vi "Request and Wait for Response.vi"(5 "headers":string, 7 "timeout in ms (-1)":i32=-1, 8 "error in":errorcluster {"code" format="Error %.0f"}, 9 "payload":string, 10 "subject":string, 11 "NATS Client in":refnum<class "NATS Client.lvclass">) -> (0 "error out":errorcluster {"code" format="Error %.0f"}, 2 "time out":bool, 3 "nats message":T1)   [LabVIEW 2020, in "NATS Client.lvlib" / "NATS Client.lvclass"]
doc: "Publishes a message and waits for a response with a blocking call."
uses:
  NATS Client.lvclass
  NATS Client.lvclass/NATS Client.ctl
  NATS Subscription/NATS Subscription.lvclass/NATS Subscription.ctl
  <vilib>/NATS/NATS Core/NATS Core.lvlib
  NATS Subscription/NATS Subscription.lvclass
  <vilib>/NATS/NATS Core/VIs/NATS HPUB.vi
  <vilib>/NATS/NATS Core/Controls/msg type.ctl
  <vilib>/NATS/NATS Core/Controls/nats message.ctl
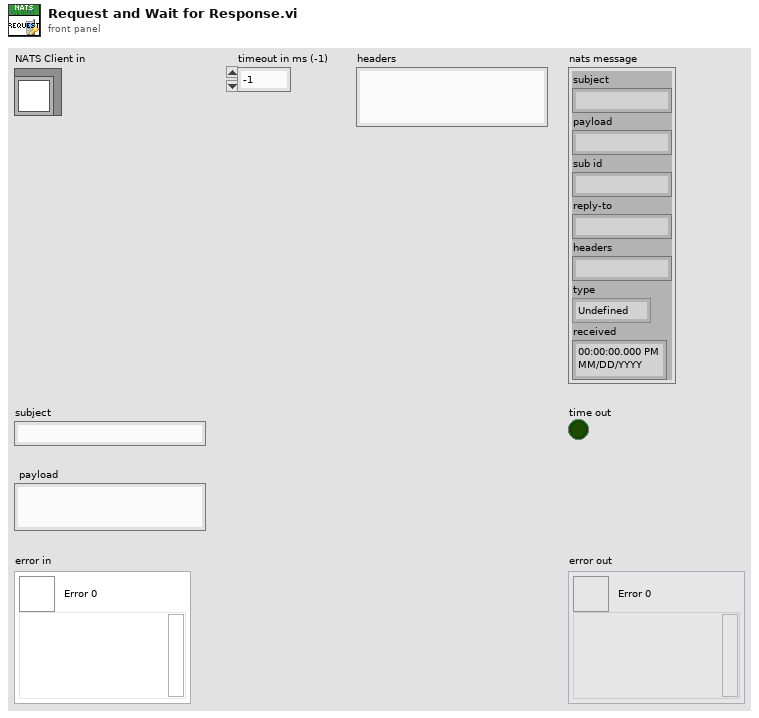
[diagram p1: front panel]
types:
  T1 = typedef "NATS Core.lvlib/nats message.ctl" = cluster{"subject":string, "payload":string, "sub id":string, "reply-to":string, "headers":string, "type":T2, "received":timestamp}
  T2 = typedef "NATS Core.lvlib/msg type.ctl" = enum16{"Undefined", "MSG", "HMSG", "+OK", "PING", "PONG", "-ERR", "INFO"}
  T3 = typedef "NATS Client.lvlib/NATS Client.lvclass/Subscription Map.ctl" = map{string, refnum<class "NATS Subscription.lvclass">}
  T4 = typedef "NATS Core.lvlib/nats connection.ctl" = cluster{"connection ID":refnum<k5>, "server INFO":string, "timeout ms":i32, "verbose?":bool, "server headers?":bool, "client headers?":bool}
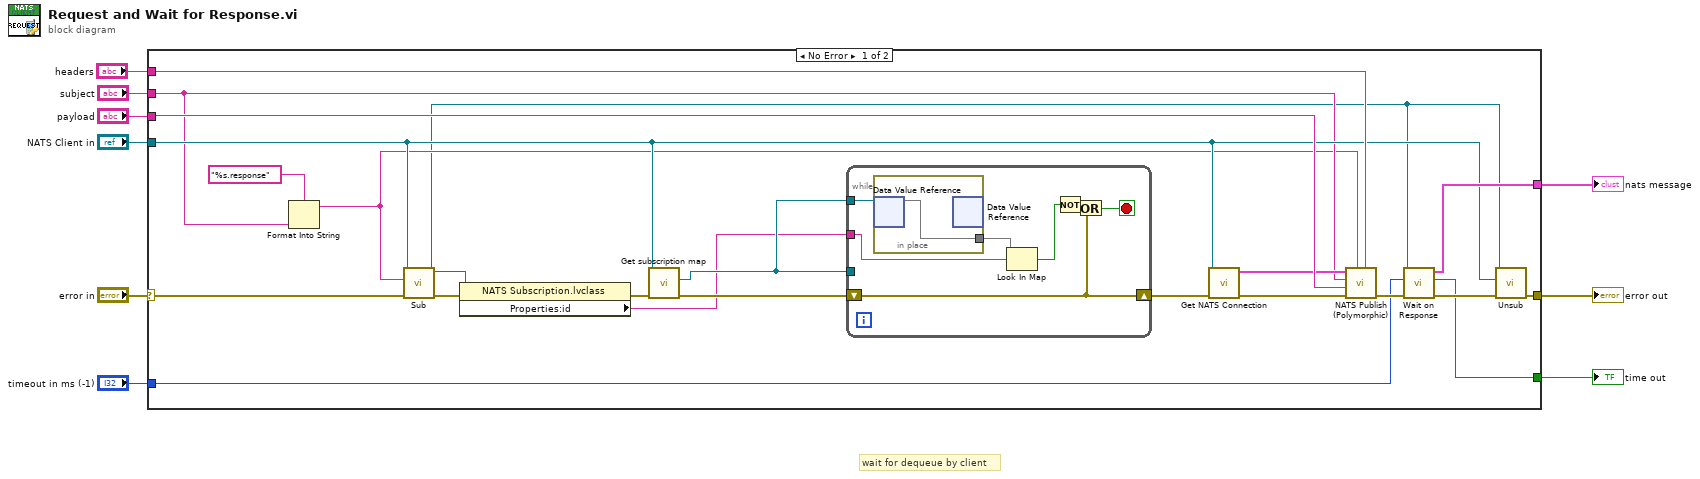
[diagram p0: block diagram]
diagram:
  # "wait for dequeue by client"
  n1 = case shown="No Error" "error in" {
    selector: "error in" -> [w28 w40]
    tunnel: [w29 w40] -> w8
    tunnel: "NATS Client in" -> [w19 _]
    tunnel: "payload" -> [w27 _]
    tunnel: "subject" -> [w14 _]
    tunnel: [w25 _] -> w4
    tunnel: "timeout in ms (-1)" -> [w26 _]
    tunnel: [w24 _] -> w2
    tunnel: "headers" -> [w20 _]
    frame No Error {
      n2 = Format Into String(format string="%s.response", w14) -> (resulting string=w12:string)  [unwired: 2 in, 1 out]
      n3 = call "Sub.vi"("error in"=w28, "subject"=w12, "NATS Client"=w19) -> ("error out"=w23:errorcluster, "NATS Subscription"=w10:refnum<class "NATS Subscription.lvclass">)  [unwired: 7 in]
      n4 = property class="NATS Subscription.lvclass"(reference=w10, error in=w23) -> (error out=w13:errorcluster, "Properties:id"=w11:string)  [unwired: 1 out]
      n5 = call "Get subscription map.vi"("error in (no error)"=w13, "NATS Client in"=w19) -> ("error out"=w18:errorcluster, "subscription map"=w16:refnum<data-value>)  [unwired: 7 in, 1 out]
      n6 = while {
        tunnel: w16 -> [_]
        shift-right: [w34] -> w17
        shift-left: w18 -> [w34]
        tunnel: w16 -> [w38]
        tunnel: w11 -> [w37]
        stop <- w35 stop-if-true
        n7 = in-place {
          in-place-border: [w39] -> w36
          n8 = in-place-dvr #1(w38) -> (w39:T3)  [unwired: 1 out]
          n9 = in-place-dvr #1() -> ()  [unwired: 1 in, 2 out]
        }
        n10 = Look In Map(map=w36, key=w37) -> (key not found?=w33:bool)  [unwired: 1 in, 1 out]
        n11 = Not(x=w33) -> (.not. x?=w32:bool)
        n12 = Or(x=w32, y=w34) -> (x .or. y?=w35:bool)
      }
      n13 = call "Get NATS Connection.vi"("error in"=w17, "NATS Client.lvlib:NATS Client.lvclass"=w19) -> ("error out"=w22:errorcluster, "NATS Connection"=w21:T4)  [unwired: 8 in]
      n14 = call-poly <vilib>:"NATS Publish (Polymorphic).vi"("headers"=w20, "reply-to"=w12, "error in"=w22, "payload"=w27, "subject"=w14, "nats connection in"=w21) -> ("error out"=w31:errorcluster)  [unwired: 4 in, 1 out]
      n15 = call "Wait on Response.vi"("error in"=w31, "timeout in ms (-1)"=w26, "NATS Subscriber in"=w10) -> ("error out"=w30:errorcluster, "time out"=w24:bool, "nats message"=w25:T1)  [unwired: 6 in]
      n16 = call "Unsub.vi"("error in"=w30, "NATS Client"=w19, "NATS Subscription"=w10) -> ("error out"=w29:errorcluster)  [unwired: 7 in, 1 out]
    }
    frame Error {
    }
  }
  "error out" <- w8
  "nats message" <- w4
  "time out" <- w2
